vi "heat alarm.vi"() -> ()   [LabVIEW 2017]
panel:
  out "look me":string
  out "moderate":bool
  out "warm":bool
  out "freez":bool
  in  "min temp":dbl
  in  "max temp":dbl
  in  "current temp":dbl
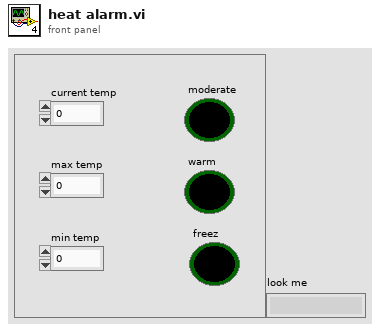
[diagram p1: front panel]
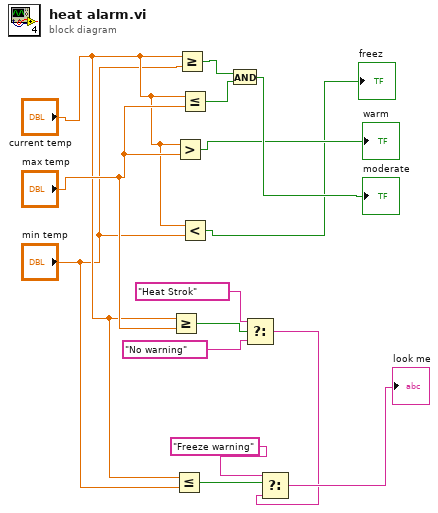
[diagram p0: block diagram]
diagram:
  n1 = Greater Or Equal?(x="current temp", y="max temp") -> (x >= y?=w7:bool)
  n2 = Less Or Equal?(x="current temp", y="min temp") -> (x <= y?=w5:bool)
  n3 = Greater?(x="current temp", y="max temp") -> (0:→"warm":bool)
  n4 = Greater Or Equal?(x="current temp", y="min temp") -> (x >= y?=w14:bool)
  n5 = Less Or Equal?(x="current temp", y="max temp") -> (x <= y?=w15:bool)
  n6 = Less?(x="current temp", y="min temp") -> (x < y?=→"freez":bool)
  n7 = And(x=w14, y=w15) -> (x .and. y?=→"moderate":bool)
  n8 = Select(t="Heat Strok", s=w7, f="No warning") -> (s? t:f=w1:string)
  n9 = Select(t="Freeze warning", s=w5, f=w1) -> (s? t:f=→"look me":string)
